vi "check_threshold.vi"(0 "Schwelle Tagestemperatur (°C)":dbl(slide) scale=0.0..10.0, 1 "Schwelle Durchschnittstemperatur (°C)":dbl(slide) scale=0.0..10.0, 2 "Anzahl Tage":i8(slide) scale=0.0..10.0, 3 "Temperature":dbl(slide) scale=0.0..10.0) -> (7 "Warnung Tagestemperatur":bool, 8 "Warnung Durchschnittstemperatur":bool, 9 "Tagestemperatur (°C)":dbl, 10 "Durchschnittstemperatur (°C)":dbl)   [LabVIEW 2025]
uses:
  <vilib>/ptbypt/NI_PtbyPt.lvlib
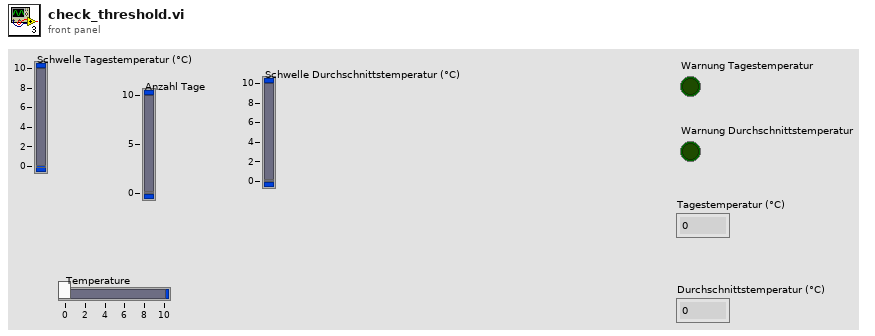
[diagram p1: front panel]
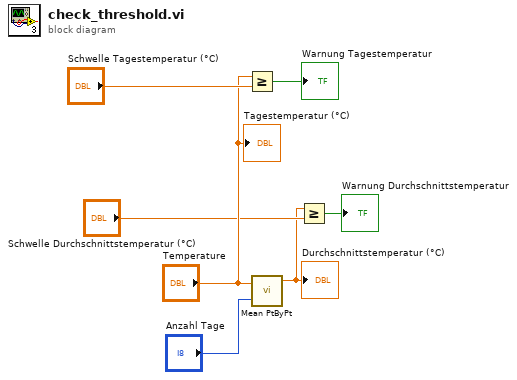
[diagram p0: block diagram]
diagram:
  n1 = Greater Or Equal?(x="Temperature", y="Schwelle Tagestemperatur (°C)") -> (x >= y?=→"Warnung Tagestemperatur":bool)
  n2 = call <vilib>:"Mean PtByPt.vi"("x"="Temperature", "sample length"="Anzahl Tage") -> ("mean"=w1:dbl)  [unwired: 2 in, 1 out]
  "Durchschnittstemperatur (°C)" <- w1
  n3 = Greater Or Equal?(x=w1, y="Schwelle Durchschnittstemperatur (°C)") -> (x >= y?=→"Warnung Durchschnittstemperatur":bool)
  "Tagestemperatur (°C)" <- "Temperature"
